vi "GVHK1Hz.vi"() -> ()   [LabVIEW 2010]
panel:
  out "Mod1Mod2Mod3/AITrapsMachs1Hz":dbl[](array[numeric])
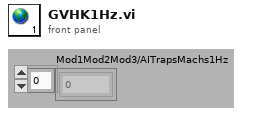
[diagram p1: front panel]
diagram:
